vi "2017-01-19 1DScanAndHold.vi"() -> ()   [LabVIEW 2016]
uses:
  <vilib>/Utility/error.llb/DialogType.ctl
  <vilib>/DAQmx/write.llb/DAQmx Write (Analog 1D DBL NChan 1Samp).vi
  <vilib>/DAQmx/write.llb/DAQmx Write (Analog DBL 1Chan 1Samp).vi
  <vilib>/DAQmx/create/channels.llb/DAQmx Create Channel (AO-Voltage-Basic).vi
  <vilib>/DAQmx/miscellaneous.llb/DAQmx Fill In Error Info.vi
panel:
  in  "Min Voltage":dbl=-10.0
  in  "Max Voltage":dbl=10.0
  in  "Output Voltage":dbl[](array[numeric])
  in  "Wait Time (ms)":dbl=100.0
  in  "Mode":enum32{"Hold", "Scan"}(radio)
  in  "Stop":bool
  in  "Physical Channel(s)":tag="Dev1/ao0"
  out "Next Voltage":dbl
  out "Current Voltage":dbl
  in  "Voltage Step":dbl=0.1
  in  "Physical Channel(s)":tag="Dev1/ao0"
  in  "Min Voltage Voltage":dbl=-10.0
  in  "Max Voltage":dbl=10.0
  # "Hold"
  # "Scan"
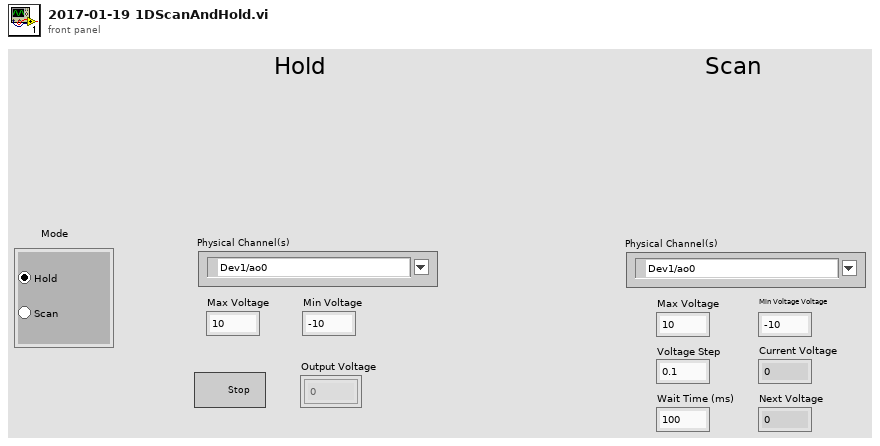
[diagram p1: front panel]
types:
  T1 = typedef "DialogType.ctl" = u16
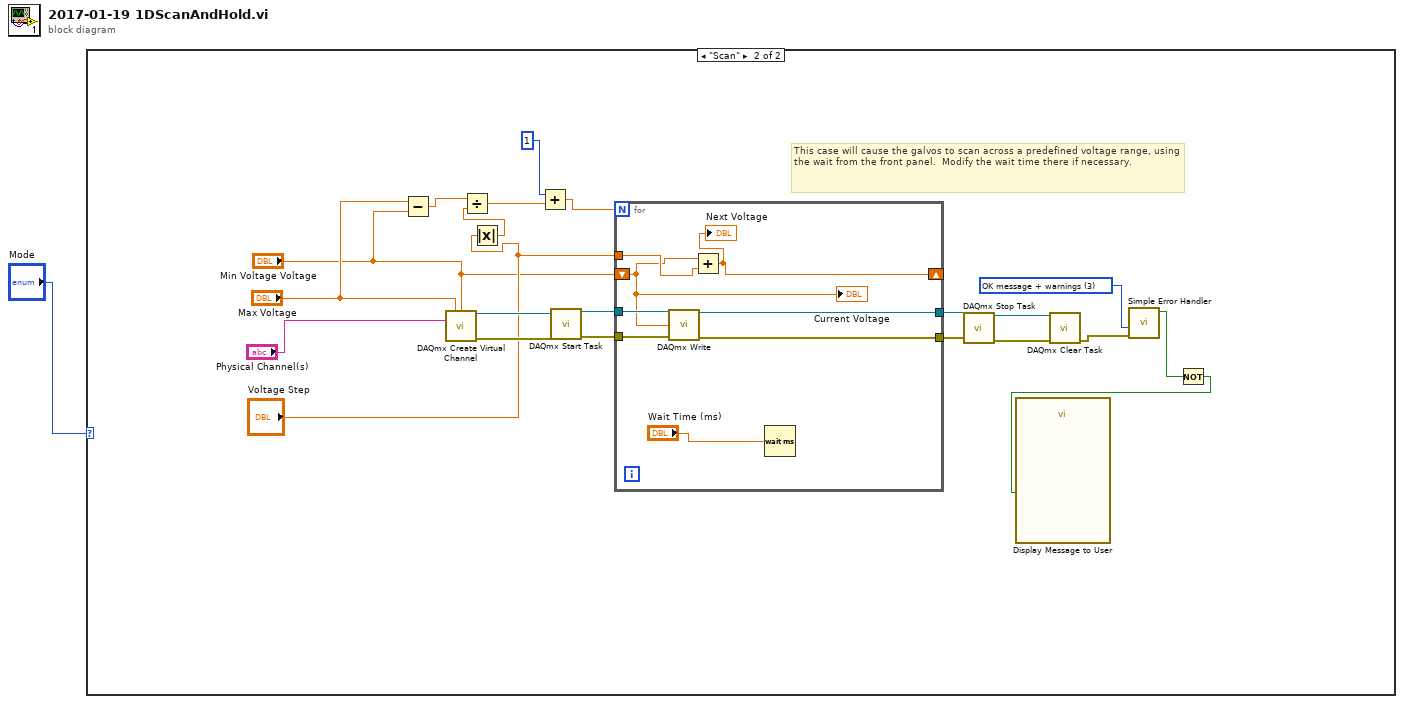
[diagram p0: block diagram]
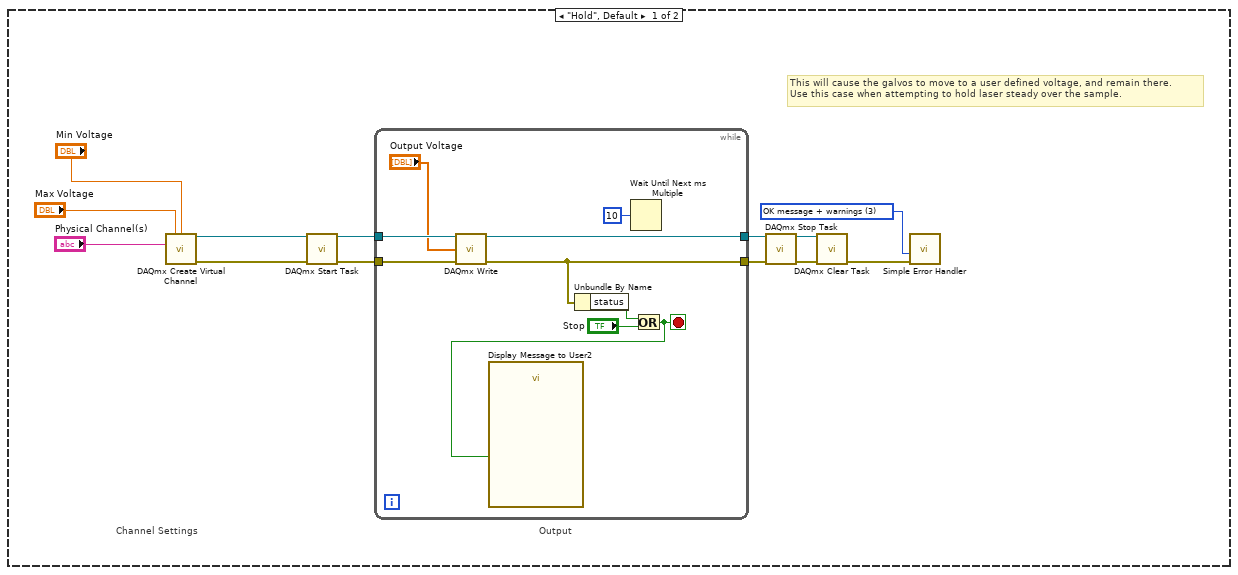
[diagram p2: hidden frame]
diagram:
  n1 = case shown="\"Scan\"" "Mode" {
    frame "Hold", Default {
      w4 = T1 3 items=["no dialog", "OK message", "continue or stop message", "OK message + warnings", "continue/stop + warnings"] ("type of dialog (OK msg:1)")
      # "This will cause the galvos to move to a user defined voltage, and remain there.\nUse this case when attempting to hold laser steady over the sample."
      # "Output"
      # "Channel Settings"
      n2 = call-poly <vilib>:"DAQmx Create Virtual Channel.vi"("maximum value"="Max Voltage", "minimum value"="Min Voltage", "physical channels"="Physical Channel(s)") -> ("task out"=w12:refnum<k21>, "error out"=w11:errorcluster)  [unwired: 11 in]
      n3 = call <vilib>:"DAQmx Start Task.vi"("task/channels in"=w12, "error in"=w11) -> ("task out"=w10:refnum<k21>, "error out"=w9:errorcluster)  [unwired: 12 in]
      n4 = while {
        tunnel: w10 -> [w23]
        tunnel: w9 -> [w22]
        tunnel: [w17] -> w7
        tunnel: [w21] -> w8
        stop <- w15 stop-if-true
        n5 = call-poly <vilib>:"DAQmx Write.vi"("task/channels in"=w23, "data"="Output Voltage", "error in"=w22) -> ("task out"=w21:refnum<k21>, "error out"=w17:errorcluster)  [unwired: 10 in, 1 out]
        n6 = Unbundle By Name(w17) -> ("status"=w19:bool)
        n7 = Wait Until Next ms Multiple(millisecond multiple=u32 10) -> ()  [unwired: 1 out]
        n8 = Or(x=w19, y="Stop") -> (x .or. y?=w15:bool)
        n9 = call "Display Message to User2"("Enable"=w15) -> ()  [unwired: 9 in, 2 out]
      }
      n10 = call <vilib>:"DAQmx Stop Task.vi"("task/channels in"=w8, "error in"=w7) -> ("task out"=w6:refnum<k21>, "error out"=w5:errorcluster)  [unwired: 12 in]
      n11 = call <vilib>:"DAQmx Clear Task.vi"("task in"=w6, "error in"=w5) -> ("error out"=w14:errorcluster)  [unwired: 13 in]
      n12 = call <vilib>:"Simple Error Handler.vi"("type of dialog (OK msg:1)"=w4, "error in (no error)"=w14) -> ()  [unwired: 3 in, 5 out]
    }
    frame "Scan" {
      w35 = T1 3 items=["no dialog", "OK message", "continue or stop message", "OK message + warnings", "continue/stop + warnings"] ("type of dialog (OK msg:1)")
      # "This case will cause the galvos to scan across a predefined voltage range, using the wait from the front panel.  Modify the wait time there if necessary."
      n13 = Subtract(x="Max Voltage", y="Min Voltage Voltage") -> (x-y=w32:dbl)
      n14 = call-poly <vilib>:"DAQmx Create Virtual Channel.vi"("maximum value"="Max Voltage", "minimum value"="Min Voltage Voltage", "physical channels"="Physical Channel(s)") -> ("task out"=w43:refnum<k21>, "error out"=w42:errorcluster)  [unwired: 11 in]
      n15 = Absolute Value(x="Voltage Step") -> (abs(x)=w30:dbl)
      n16 = Divide(x=w32, y=w30) -> (x/y=w28:dbl)
      n17 = Add(x=1, y=w28) -> (x+y=w26:dbl)
      n18 = call <vilib>:"DAQmx Start Task.vi"("task/channels in"=w43, "error in"=w42) -> ("task out"=w41:refnum<k21>, "error out"=w40:errorcluster)  [unwired: 12 in]
      n19 = for {
        N: w26 -> [_]
        tunnel: w41 -> [w52]
        tunnel: w40 -> [w51]
        tunnel: [w50] -> w39
        tunnel: [w48] -> w38
        tunnel: "Voltage Step" -> [w49]
        shift-right: [w46] -> _
        shift-left: "Min Voltage Voltage" -> [w47]
        n20 = call-poly <vilib>:"DAQmx Write.vi"("task/channels in"=w52, "data"=w47, "error in"=w51) -> ("task out"=w48:refnum<k21>, "error out"=w50:errorcluster)  [unwired: 10 in, 1 out]
        n21 = Add(x=w47, y=w49) -> (x+y=w46:dbl)
        "Next Voltage" <- w46
        n22 = Wait (ms)(milliseconds to wait="Wait Time (ms)") -> ()  [unwired: 1 out]
        "Current Voltage" <- w47
      }
      n23 = call <vilib>:"DAQmx Stop Task.vi"("task/channels in"=w38, "error in"=w39) -> ("task out"=w36:refnum<k21>, "error out"=w37:errorcluster)  [unwired: 12 in]
      n24 = call <vilib>:"DAQmx Clear Task.vi"("task in"=w36, "error in"=w37) -> ("error out"=w34:errorcluster)  [unwired: 13 in]
      n25 = call <vilib>:"Simple Error Handler.vi"("type of dialog (OK msg:1)"=w35, "error in (no error)"=w34) -> ("error?"=w25:bool)  [unwired: 3 in, 4 out]
      n26 = Not(x=w25) -> (.not. x?=w24:bool)
      n27 = call "Display Message to User"("Enable"=w24) -> ()  [unwired: 9 in, 2 out]
    }
  }
